vi "太阳能控制器MPPT12.vi"() -> ()   [LabVIEW 2016, in "环境动力监测库.lvlib"]
uses:
  <vilib>/Utility/miscctls.llb/LVPointTypeDef.ctl
  <vilib>/Utility/config.llb/NI_LVConfig.lvlib
  <vilib>/ptbypt/NI_PtbyPt.lvlib
panel:
  out "x+1":u32
  in  "解除告警":bool
  out "串口":string
  in  "串口启用":bool
  in  "报警设置":bool
  in  "MPPT-12 串口":refnum<visa-resource-name> caption="MPPT-12"
  out "状态":string
  out "充放电信息":T1 caption="充放电信息_KWH" {"总累计充电量" format="%.2f"; "当年累计充电量" format="%.2f"; "当月累计充电量" format="%.2f"; "当日累计充电量" format="%.2f"; "当年累计用电量" format="%.2f"; "当月累计用电量" format="%.2f"; "当日累计用电量" format="%.2f"}
  out "通信":bool=TRUE
  out "控制器信息":cluster{"设备温度":dbl}
  out "直流负载信息":cluster{"负载电压":dbl, "负载电流":dbl, "负载功率":dbl}
  out "蓄电池信息":T2
  out "阵列信息":cluster{"阵列电压":dbl, "阵列电流":dbl, "发电功率":dbl}
  # "太阳能控制器MPPT-12"
  # "kW·h"
  # "kW·h"
  # "kW·h"
  # "kW·h"
  # "kW·h"
  # "kW·h"
  # "kW·h"
  # "kW·h"
  # "℃"
  # "V"
  # "A"
  # "W"
  # "V"
  # "A"
  # "V"
  # "A"
  # "℃"
  # "%"
  # "V"
  # "A"
  # "W"
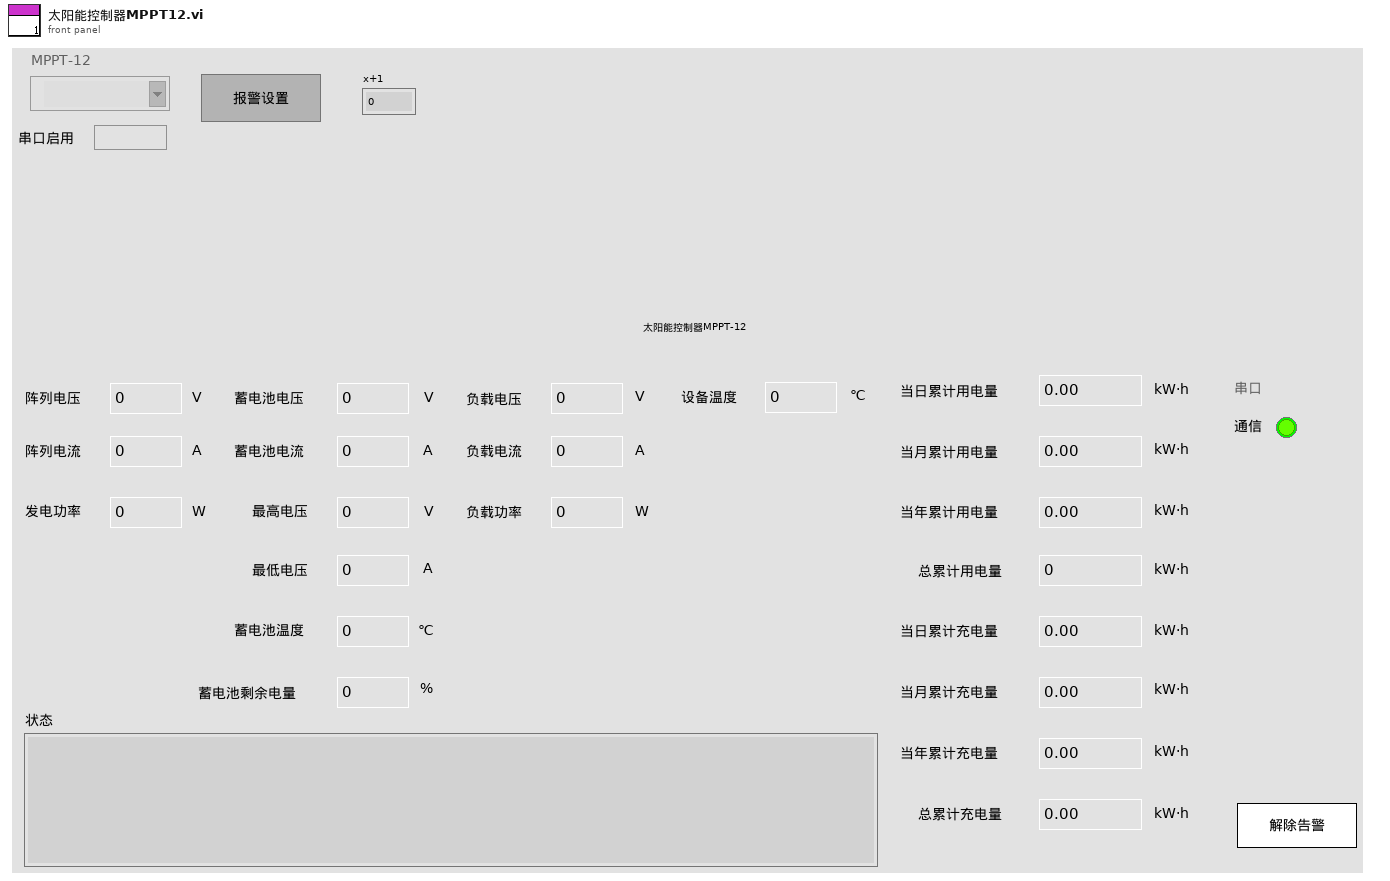
[diagram p1: front panel]
types:
  T1 = cluster{"当日累计用电量":sgl, "当月累计用电量":sgl, "当年累计用电量":sgl, "总累计用电量":sgl, "当日累计充电量":sgl, "当月累计充电量":sgl, "当年累计充电量":sgl, "总累计充电量":sgl}
  T2 = cluster{"蓄电池电压":dbl, "蓄电池电流":dbl, "最高电压":dbl, "最低电压":dbl, "蓄电池温度":dbl, "蓄电池剩余电量":dbl}
  T3 = cluster{"baud rate (bps)":u32, "stop bits":u16, "parity":u16, "flow control":u16, "timeout":u32, "retries":i32}
  T4 = cluster{"监测项描述:输出":string, "连接方式":enum16{"串口", "TCP"}, "端口":string, "IP address:":string, "Port:":string, "站号":u64, "传感器型号":string, "波特率":u64, "data bits":u64, "停止位":u16, "奇偶校验":u16, "声光告警启用":bool}
  T5 = typedef "LVPointTypeDef.ctl" = cluster{"Horizontal":i16, "Vertical":i16}
  T6 = cluster{"漏水监测输出":cluster{"漏水监测告警":bool, "告警内容":string}, "门禁监测输出":cluster{"门禁监测告警":bool, "告警内容":string}, "门禁监测输出2":cluster{"门禁监测告警":bool, "告警内容":string}, "温湿度监测输出":cluster{"温湿度监测告警":bool, "告警内容":string}, "烟雾监测输出":cluster{"烟雾监测告警":bool, "告警内容":string}, "空调监测输出":cluster{"空调监测告警":bool, "告警内容":string}, "自动重合闸输出":cluster{"自动重合闸告警":bool, "告警内容":string}, "红外入侵输出":cluster{"红外入侵告警":bool, "告警内容":string}, "振动输出":cluster{"振动告警":bool, "告警内容":string}, "UPS输出":cluster{"UPS告警":bool, "告警内容":string}, "蓄电池输出":cluster{"蓄电池告警":bool, "告警内容":string}, "蓄电池输出2":cluster{"蓄电池告警":bool, "告警内容":string}, "GPS输出":cluster{"定位告警":bool, "告警内容":string}, "北斗输出":cluster{"定位告警":bool, "告警内容":string}, "气象输出":cluster{"气象告警":bool, "告警内容":string}, "废液输出":cluster{"废液告警":bool, "告警内容":string}, "废液输出2":cluster{"废液告警":bool, "告警内容":string}}
  T7 = cluster{"时间":timestamp, "阵列电压_V":dbl, "阵列电流_A":dbl, "发电功率_W":dbl, "蓄电池电压_V":dbl, "蓄电池电流_A":dbl, "最高电压_V":dbl, "最低电压_A":dbl, "蓄电池温度_℃":dbl, "蓄电池剩余电量_%":dbl, "负载电压_V":dbl, "负载电流_A":dbl, "负载功率_W":dbl, "设备温度_℃":dbl, "当日累计用电量_KWH":dbl, "当月累计用电量_KWH":dbl, "当年累计用电量_KWH":dbl, "总累计用电量_KWH":dbl, "当日累计充电量_KWH":dbl, "当月累计充电量_KWH":dbl, "当年累计充电量_KWH":dbl, "总累计充电量_KWH":dbl}
  T8 = typedef "LVDateTimeRec.ctl" = cluster{"秒数的小数部分":dbl, "秒":i32, "分":i32, "时":i32, "日":i32, "月":i32, "年":i32, "天数（周）":i32, "天数（年）":i32, "DST":i32}
  T9 = cluster{"市电":cluster{"状态":bool, "电压:":u16, "电流：":dbl, "详情  ":bool}, "UPS":cluster{"状态":bool, "输入电压:":sgl, "输出电压:":sgl, "电池电量:":u8, "电量":u16, "详情  ":bool}, "蓄电池12V":cluster{"状态":bool, "电压:":sgl, "电流:":sgl, "电池电量:":u8, "电量":u16, "详情  ":bool}, "蓄电池24V":cluster{"状态":bool, "电压:":sgl, "电流:":sgl, "电池电量:":u8, "电量":u16, "详情  ":bool}}
  T10 = cluster{"状态":cluster{"蓄电池状态":string, "阵列状态":string, "充电状态":string, "负载状态":string, "设备状态":string}, "充放电信息":cluster{"当日累计用电量":sgl, "当月累计用电量":sgl, "当年累计用电量":sgl, "总累计用电量":sgl, "当日累计充电量":sgl, "当月累计充电量":sgl, "当年累计充电量":sgl, "总累计充电量":sgl}, "控制器信息":cluster{"设备温度℃":dbl}, "蓄电池信息":cluster{"蓄电池电压V":dbl, "蓄电池电流A":dbl, "最高电压V":dbl, "最低电压A":dbl, "蓄电池温度℃":dbl, "蓄电池剩余电量%":dbl}, "阵列信息":cluster{"阵列电压V":dbl, "阵列电流A":dbl, "发电功率W":dbl}, "直流负载信息":cluster{"负载电压V":dbl, "负载电流A":dbl, "负载功率W":dbl}, "error out":errorcluster}
  T11 = enum32{"Bad", "Idle", "Run top level", "Running"}
  T12 = typedef "NI_LVConfig.lvlib/Config Data RefNum.ctl" = refnum<k1>
  T13 = enum8{"Enabled", "Disabled", "Disabled and Grayed Out"}
  T14 = cluster{"蓄电池电压V":dbl, "蓄电池电流A":dbl, "最高电压V":dbl, "最低电压A":dbl, "蓄电池温度℃":dbl, "蓄电池剩余电量%":dbl}
  T15 = cluster{"蓄电池状态":string, "阵列状态":string, "充电状态":string, "负载状态":string, "设备状态":string}
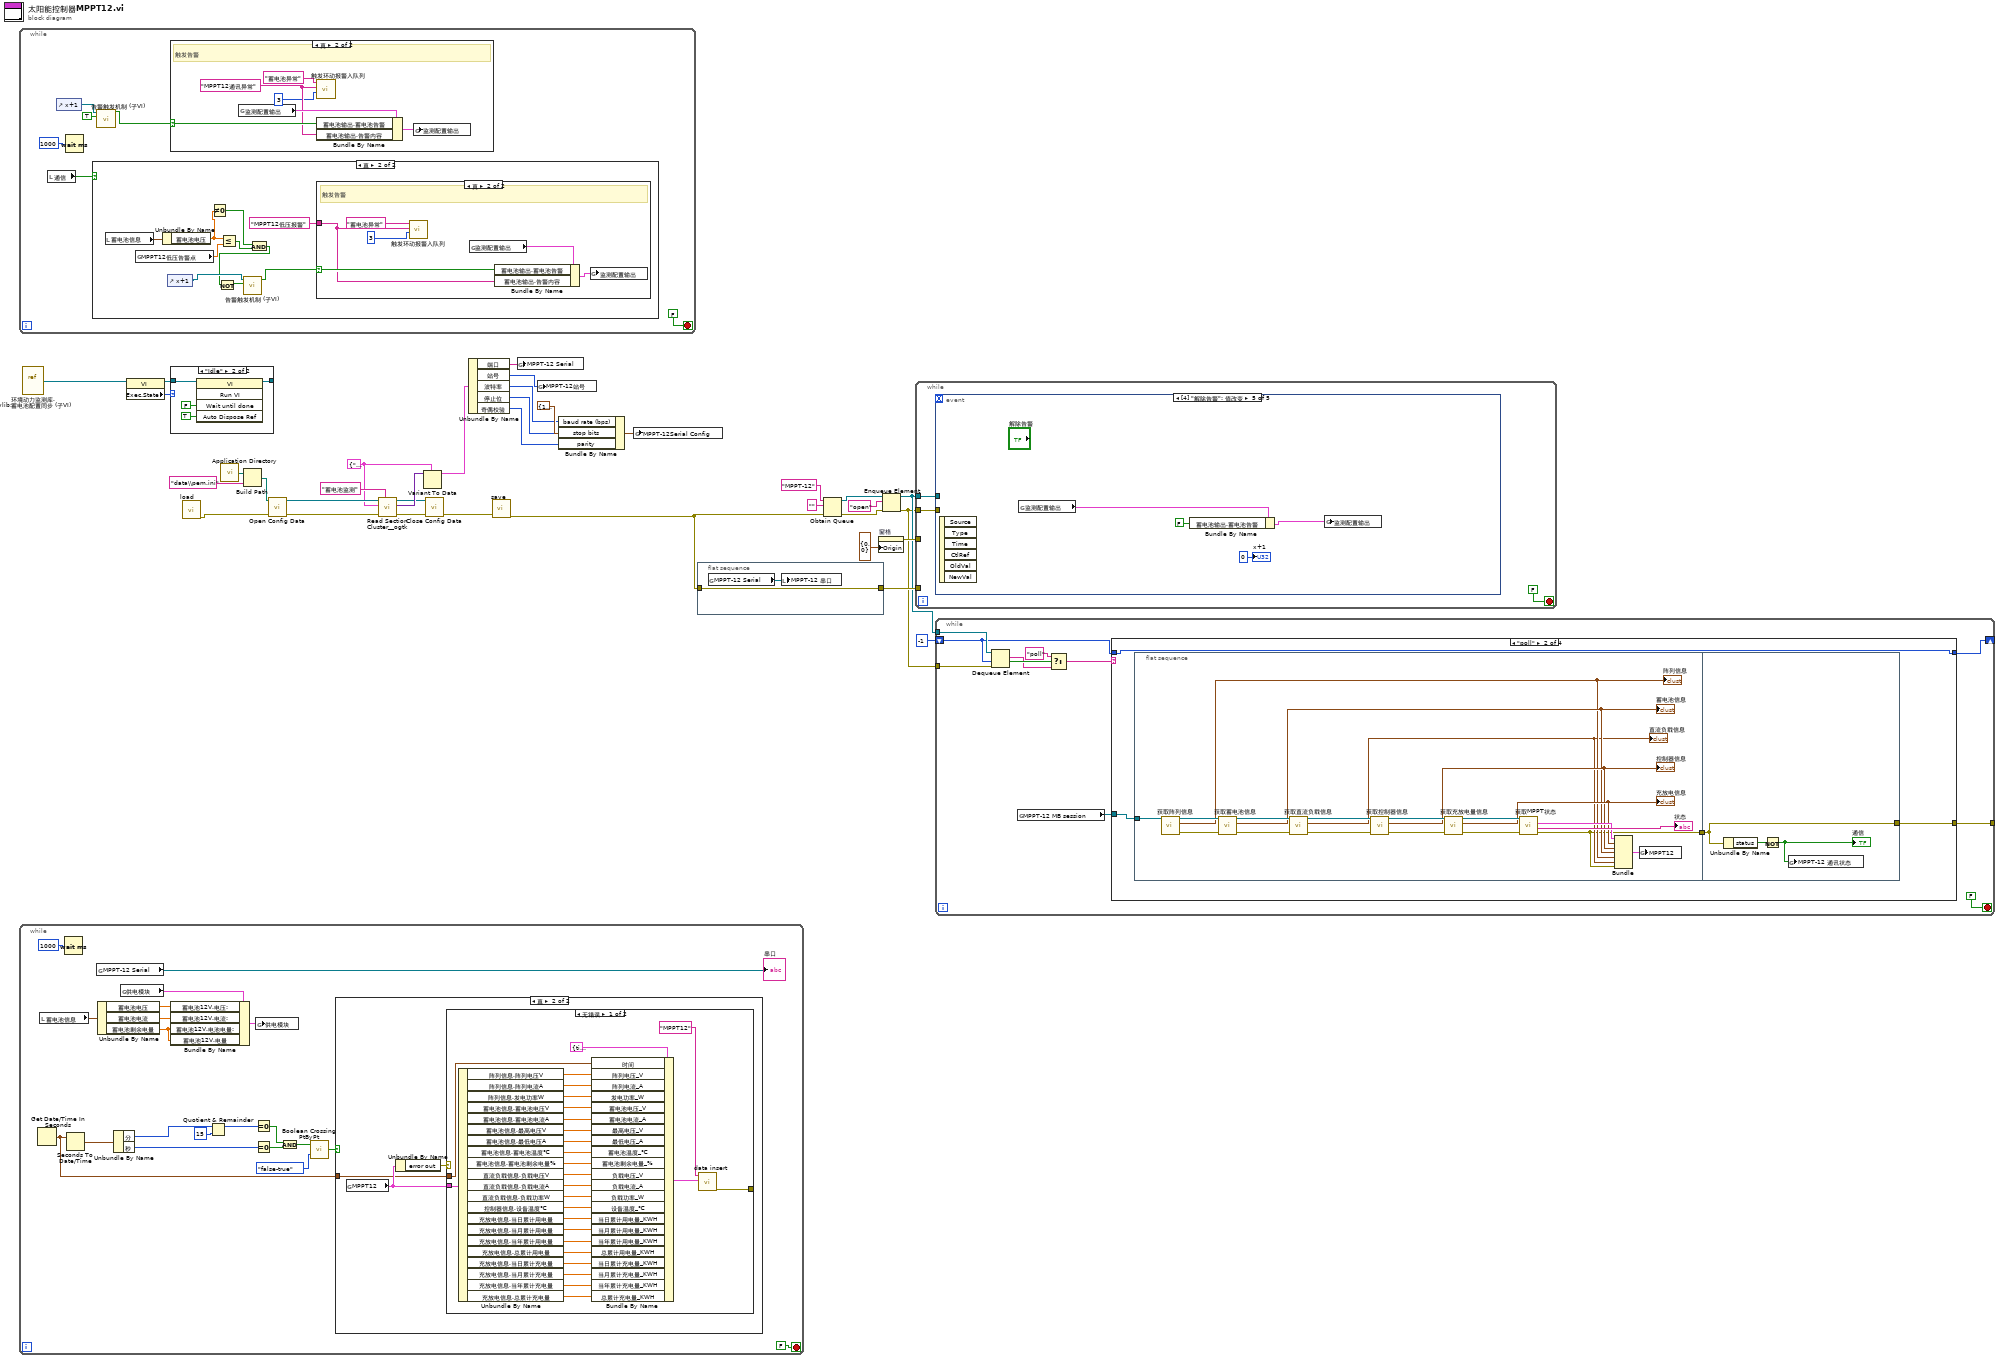
[diagram p0: block diagram]
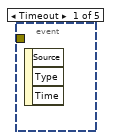
[diagram p8: hidden frame]
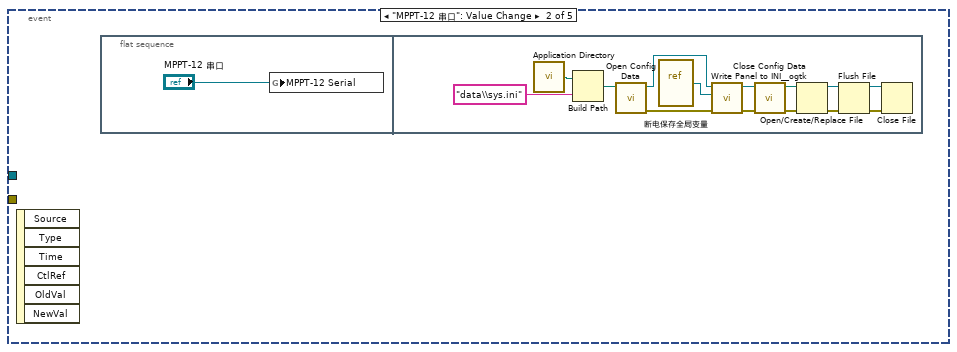
[diagram p9: hidden frame]
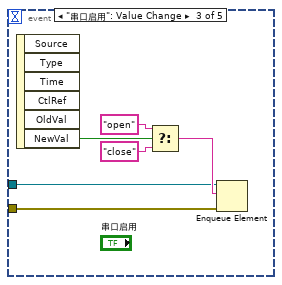
[diagram p10: hidden frame]
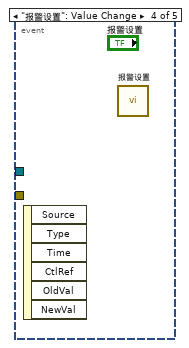
[diagram p11: hidden frame]
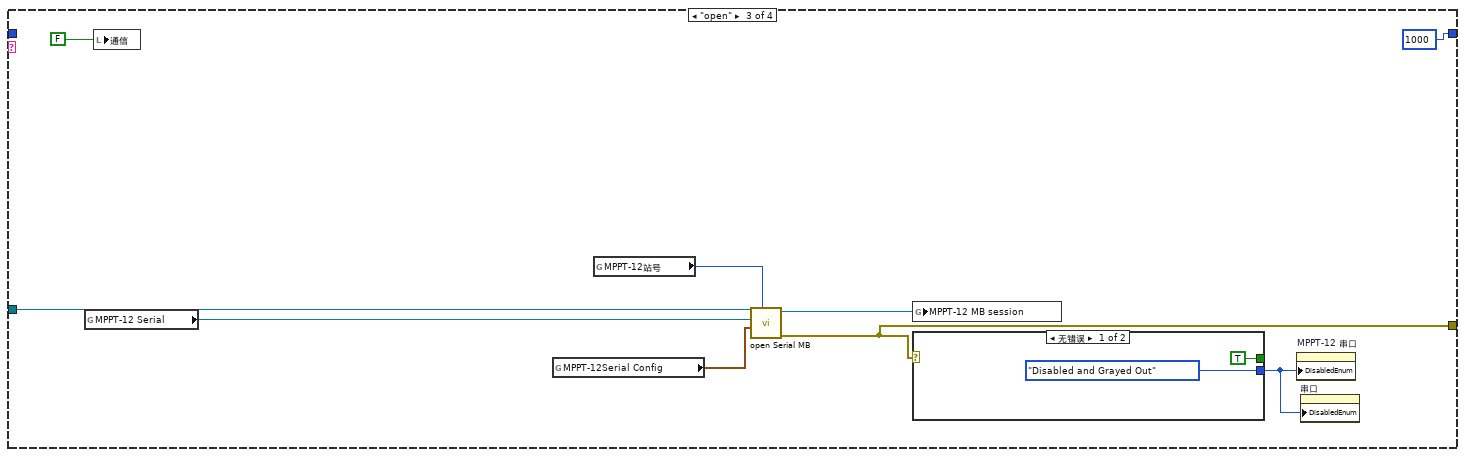
[diagram p13: hidden frame]
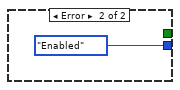
[diagram p14: hidden frame]
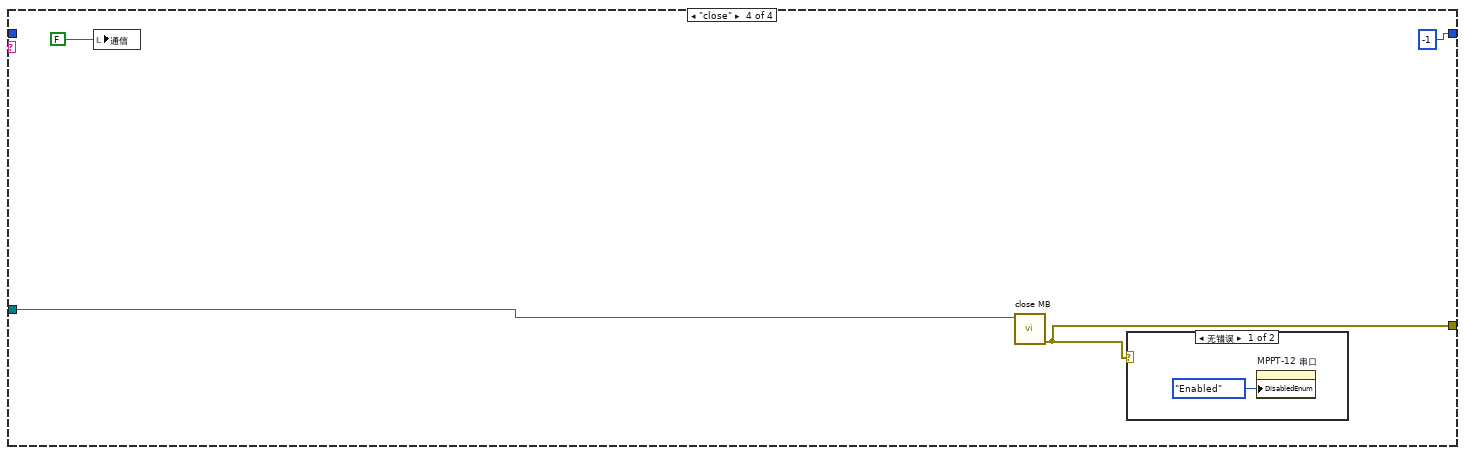
[diagram p15: hidden frame]
diagram:
  w14 = T4 {"监测项描述:输出"="", "连接方式"=enum."串口", "端口"="", "IP address:"="", "Port:"="", "站号"=19200, "传感器型号"="", "波特率"=19200, "data bits"=8, "停止位"=10, "奇偶校验"=0, "声光告警启用"=FALSE} ("输入簇")
  n1 = while {
    stop <- FALSE stop-if-true
    n2 = local read "通信"() -> (w39:bool)
    n3 = control-ref of="x+1"() -> (w38:refnum<vi>)
    n4 = Wait (ms)(milliseconds to wait=u32 1000 ("等待时间（毫秒）")) -> ()  [unwired: 1 out]
    n5 = case shown="真" w39 {
      frame False {
      }
      frame True {
        n6 = local read "蓄电池信息"() -> (w57:T2)
        n7 = global read "断电保存全局变量.vi" "MPPT12低压告警点"() -> (w56:dbl)
        n8 = Unbundle By Name(w57) -> ("蓄电池电压"=w50:dbl)
        n9 = control-ref of="x+1"() -> (w52:refnum<vi>)
        n10 = Not Equal To 0?(x=w50) -> (x != 0?=w49:bool)
        n11 = Less Or Equal?(x=w50, y=w56) -> (x <= y?=w51:bool)
        n12 = And(x=w49, y=w51) -> (x .and. y?=w48:bool)
        n13 = Not(x=w48) -> (.not. x?=w54:bool)
        n14 = call "告警触发机制 (子VI).vi"("状态输出"=w54, "Digital输入"=w52) -> ("触发告警"=w53:bool)  [unwired: 8 in, 1 out]
        n15 = case shown="真" w53 {
          selector: w53 -> [_ w63]
          tunnel: "MPPT12低压报警" ("设备") -> [_ w59]
          frame False {
          }
          frame True {
            # "触发告警"
            n16 = call "触发环动报警入队列.vi"("code"=3, "备注"=w59, "报警内容"="蓄电池异常" ("设备")) -> ()  [unwired: 9 in]
            n17 = global read "内部交互全局变量.vi" "监测配置输出"() -> (w62:T6)
            n18 = Bundle By Name(cluster=w62, "蓄电池输出.蓄电池告警"=w63, "蓄电池输出.告警内容"=w59) -> (w61:T6)
            n19 = global write "内部交互全局变量.vi" "监测配置输出"(w61) -> ()
          }
        }
      }
    }
    n20 = call "告警触发机制 (子VI).vi"("状态输出"=TRUE, "Digital输入"=w38) -> ("触发告警"=w37:bool)  [unwired: 8 in, 1 out]
    n21 = case shown="真" w37 {
      selector: w37 -> [_ w47]
      frame False {
      }
      frame True {
        w43 = "MPPT12通讯异常" ("报警内容")
        # "触发告警"
        n22 = global read "内部交互全局变量.vi" "监测配置输出"() -> (w46:T6)
        n23 = call "触发环动报警入队列.vi"("code"=3, "备注"=w43, "报警内容"="蓄电池异常" ("设备")) -> ()  [unwired: 9 in]
        n24 = Bundle By Name(cluster=w46, "蓄电池输出.蓄电池告警"=w47, "蓄电池输出.告警内容"=w43) -> (w45:T6)
        n25 = global write "内部交互全局变量.vi" "监测配置输出"(w45) -> ()
      }
    }
  }
  n26 = while {
    stop <- FALSE stop-if-true
    n27 = Get Date/Time In Seconds() -> (seconds since 1Jan1904=w71:timestamp)
    n28 = local read "蓄电池信息"() -> (w67:T2)
    n29 = Wait (ms)(milliseconds to wait=u32 1000 ("等待时间（毫秒）")) -> ()  [unwired: 1 out]
    n30 = Seconds To Date/Time(time stamp (now)=w71) -> (date time rec=w81:T8)  [unwired: 1 in]
    n31 = global read "断电保存全局变量.vi" "MPPT-12 Serial"() -> (→"串口":refnum<visa-resource-name>)
    n32 = Unbundle By Name(w67) -> ("蓄电池电压"=w66:dbl, "蓄电池电流"=w65:dbl, "蓄电池剩余电量"=w64:dbl)
    n33 = Unbundle By Name(w81) -> ("分"=w80:i32, "秒"=w77:i32)
    n34 = global read "内部交互全局变量.vi" "供电模块"() -> (w69:T9)
    n35 = Bundle By Name(cluster=w69, "蓄电池12V.电压:"=w66, "蓄电池12V.电流:"=w65, "蓄电池12V.电池电量:"=w64, "蓄电池12V.电量"=w64) -> (w68:T9)
    n36 = Quotient & Remainder(x=w80, y=15) -> (x-y*floor(x/y)=w78:i32)  [unwired: 1 out]
    n37 = Equal To 0?(x=w78) -> (x = 0?=w76:bool)
    n38 = Equal To 0?(x=w77) -> (x = 0?=w75:bool)
    n39 = global write "内部交互全局变量.vi" "供电模块"(w68) -> ()
    n40 = And(x=w76, y=w75) -> (x .and. y?=w74:bool)
    n41 = call <vilib>:"Boolean Crossing PtByPt.vi"("direction"=enum16{"either", "false-true", "true-false"}."false-true", "input"=w74) -> ("crossing"=w72:bool)  [unwired: 1 in]
    n42 = case shown="真" w72 {
      tunnel: w71 -> [_ w84]
      frame False {
      }
      frame True {
        n43 = global read "太阳能控制器全局.vi" "MPPT12"() -> (w85:T10)
        n44 = Unbundle By Name(w85) -> ("error out"=w86:errorcluster)
        n45 = case shown="无错误" w86 {
          tunnel: w85 -> [w91 _]
          tunnel: w84 -> [w90 _]
          tunnel: [w87 _] -> _
          frame No Error {
            n46 = Unbundle By Name(w91) -> ("阵列信息.阵列电压V"=w93:dbl, "阵列信息.阵列电流A"=w94:dbl, "阵列信息.发电功率W"=w95:dbl, "蓄电池信息.蓄电池电压V"=w96:dbl, "蓄电池信息.蓄电池电流A"=w97:dbl, "蓄电池信息.最高电压V"=w98:dbl, "蓄电池信息.最低电压A"=w99:dbl, "蓄电池信息.蓄电池温度℃"=w100:dbl, "蓄电池信息.蓄电池剩余电量%"=w101:dbl, "直流负载信息.负载电压V"=w102:dbl, "直流负载信息.负载电流A"=w103:dbl, "直流负载信息.负载功率W"=w104:dbl, "控制器信息.设备温度℃"=w105:dbl, "充放电信息.当日累计用电量"=w106:sgl, "充放电信息.当月累计用电量"=w107:sgl, "充放电信息.当年累计用电量"=w108:sgl, "充放电信息.总累计用电量"=w109:sgl, "充放电信息.当日累计充电量"=w110:sgl, "充放电信息.当月累计充电量"=w111:sgl, "充放电信息.当年累计充电量"=w112:sgl, "充放电信息.总累计充电量"=w113:sgl)
            n47 = Bundle By Name(cluster=T7 {"时间"=timestamp(0 s since 1904-01-01), "阵列电压_V"=0.0, "阵列电流_A"=0.0, "发电功率_W"=0.0, "蓄电池电压_V"=0.0, "蓄电池电流_A"=0.0, "最高电压_V"=0.0, "最低电压_A"=0.0, "蓄电池温度_℃"=0.0, "蓄电池剩余电量_%"=0.0, "负载电压_V"=0.0, "负载电流_A"=0.0, "负载功率_W"=0.0, "设备温度_℃"=0.0, "当日累计用电量_KWH"=0.0, "当月累计用电量_KWH"=0.0, "当年累计用电量_KWH"=0.0, "总累计用电量_KWH"=0.0, "当日累计充电量_KWH"=0.0, "当月累计充电量_KWH"=0.0, "当年累计充电量_KWH"=0.0, "总累计充电量_KWH"=0.0} ("data in"), "时间"=w90, "阵列电压_V"=w93, "阵列电流_A"=w94, "发电功率_W"=w95, "蓄电池电压_V"=w96, "蓄电池电流_A"=w97, "最高电压_V"=w98, "最低电压_A"=w99, "蓄电池温度_℃"=w100, "蓄电池剩余电量_%"=w101, "负载电压_V"=w102, "负载电流_A"=w103, "负载功率_W"=w104, "设备温度_℃"=w105, "当日累计用电量_KWH"=w106, "当月累计用电量_KWH"=w107, "当年累计用电量_KWH"=w108, "总累计用电量_KWH"=w109, "当日累计充电量_KWH"=w110, "当月累计充电量_KWH"=w111, "当年累计充电量_KWH"=w112, "总累计充电量_KWH"=w113) -> (w89:T7)
            n48 = call "data insert.vi"("data in"=w89, "table"="MPPT12") -> ("error out"=w87:errorcluster)  [unwired: 9 in]
          }
          frame Error {
          }
        }
      }
    }
  }
  n49 = vi-ref "环境动力监测库.lvlib:蓄电池配置同步 (子VI).vi"() -> (w10:refnum<vi>)
  n50 = property class="VI"(reference=w10) -> (reference out=w11:refnum<vi>, "Exec.State"=w12:T11)  [unwired: 1 in, 1 out]
  n51 = case shown="\"Idle\"" w12 {
    tunnel: w11 -> [w114 w116]
    tunnel: [w114 w115] -> _
    frame "Bad", Default {
    }
    frame "Idle" {
      n52 = invoke class="VI" method="Run VI"(reference=w116, "Wait until done"=FALSE ("结束前等待"), "Auto Dispose Ref"=TRUE ("自动销毁引用")) -> (reference out=w115:refnum<vi>)  [unwired: 2 in, 4 out]
    }
  }
  n53 = call "load.vi"() -> ("error out"=w3:errorcluster)  [unwired: 11 in]
  n54 = call <vilib>:"Application Directory.vi"() -> ("Application Directory"=w18:path)
  n55 = Build Path(base path=w18, name or relative path="data\\pem.ini" ("名称或相对路径")) -> (appended path=w17:path)
  n56 = call <vilib>:"Open Config Data.vi"("error in (no error)"=w3, "configuration file path"=w17) -> ("error out"=w16:errorcluster, "refnum"=w15:T12)  [unwired: 7 in, 1 out]
  n57 = call <userlib>:"Read Section Cluster__ogtk.vi"("section (optional)"="蓄电池监测", "error in (no error)"=w16, "Section Formatted Cluster Type"=w14, "refnum"=w15) -> ("error out"=w22:errorcluster, "Section Formatted Cluster"=w23:variant, "dup refnum"=w21:T12)  [unwired: 3 in, 2 out]
  n58 = Variant To Data(type=w14, Variant=w23) -> (data=w24:T4)  [unwired: 1 in, 1 out]
  n59 = call <vilib>:"Close Config Data.vi"("error in (no error)"=w22, "refnum"=w21) -> ("error out"=w2:errorcluster)  [unwired: 8 in, 1 out]
  n60 = Unbundle By Name(w24) -> ("端口"=w13:string, "站号"=w7:u64, "波特率"=w6:u64, "停止位"=w5:u16, "奇偶校验"=w4:u16)
  n61 = call "save.vi"("error in (no error)"=w2) -> ("error out"=w1:errorcluster)  [unwired: 10 in]
  n62 = global write "断电保存全局变量.vi" "MPPT-12 Serial"(w13) -> ()
  n63 = global write "断电保存全局变量.vi" "MPPT-12站号"(w7) -> ()
  n64 = Bundle By Name(cluster=T3 {"baud rate (bps)"=115200, "stop bits"=10, "parity"=0, "flow control"=0, "timeout"=1000, "retries"=1} ("MPPT-24Serial Config"), "baud rate (bps)"=w6, "stop bits"=w5, "parity"=w4) -> (w8:T3)
  n65 = global write "断电保存全局变量.vi" "MPPT-12Serial Config"(w8) -> ()
  n66 = flat-sequence {
    tunnel: w1 -> [w119]
    tunnel: [w119] -> w27
    frame #0 {
      n67 = global read "断电保存全局变量.vi" "MPPT-12 Serial"() -> (w120:refnum<visa-resource-name>)
      n68 = local write "MPPT-12 串口"(w120) -> ()
    }
  }
  n69 = Obtain Queue(name (unnamed)="MPPT-12" ("名称（未命名）"), element data type="", error in (no error)=w1) -> (queue out=w29:refnum<queue>, error out=w28:errorcluster)  [unwired: 2 in, 1 out]
  n70 = property on="窗格" class="Pane"("Origin"=T5 {"Horizontal"=0, "Vertical"=0} ("原点")) -> (error out=w33:errorcluster)  [unwired: 2 in, 1 out]
  n71 = Enqueue Element(queue=w29, element="open" ("元素"), error in (no error)=w28) -> (queue out=w26:refnum<queue>, error out=w25:errorcluster)  [unwired: 1 in, 1 out]
  n72 = while {
    tunnel: w33 -> [_]
    tunnel: w27 -> [_]
    tunnel: w26 -> [w122]
    tunnel: w25 -> [w121]
    stop <- FALSE stop-if-true
    n73 = event shown="[4] \"解除告警\": 值改变" {
      selector: _ -> [_ _ _ _ _]
      dyn-events: _ -> [_ _ _ _ _]
      timeout: _ -> [_ _ _ _ _]
      tunnel: w122 -> [_ _ w140 _ _]
      tunnel: w121 -> [_ _ w139 _ _]
      event Timeout {
        n74 = event-data() -> ()  [unwired: 1 in, 3 out]
      }
      event "MPPT-12 串口": Value Change {
        n75 = event-data() -> ()  [unwired: 1 in, 6 out]
        n76 = flat-sequence {
          frame #0 {
            n77 = global write "断电保存全局变量.vi" "MPPT-12 Serial"("MPPT-12 串口") -> ()
          }
          frame #1 {
            n78 = call <vilib>:"Application Directory.vi"() -> ("Application Directory"=w138:path)
            n79 = Build Path(base path=w138, name or relative path="data\\sys.ini" ("名称或相对路径")) -> (appended path=w136:path)
            n80 = call <vilib>:"Open Config Data.vi"("configuration file path"=w136) -> ("error out"=w132:errorcluster, "refnum"=w135:T12)  [unwired: 8 in, 1 out]
            n81 = vi-ref "断电保存全局变量.vi"() -> (w134:refnum<vi>)
            n82 = call <userlib>:"Write Panel to INI__ogtk.vi"("error in (no error)"=w132, "VI ref"=w134, "refnum"=w135) -> ("error out"=w131:errorcluster, "refnum out"=w133:T12)  [unwired: 7 in]
            n83 = call <vilib>:"Close Config Data.vi"("error in (no error)"=w131, "refnum"=w133) -> ("error out"=w126:errorcluster, "file path"=w125:path)  [unwired: 8 in]
            n84 = Open/Create/Replace File(file path (use dialog)=w125, error in=w126) -> (refnum out=w129:refnum<file>, error out=w130:errorcluster)  [unwired: 4 in, 1 out]
            n85 = Flush File(refnum=w129, error in=w130) -> (refnum out=w128:refnum<file>, error out=w127:errorcluster)
            n86 = Close File(refnum=w128, error in=w127) -> ()  [unwired: 2 out]
          }
        }
      }
      event "串口启用": Value Change {
        n87 = event-data() -> ("NewVal"=w141:bool)  [unwired: 1 in, 5 out]
        n88 = Select(t="open", s=w141, f="close") -> (s? t:f=w143:string)
        n89 = Enqueue Element(queue=w140, element=w143, error in (no error)=w139) -> ()  [unwired: 1 in, 3 out]
      }
      event "报警设置": Value Change {
        n90 = event-data() -> ()  [unwired: 1 in, 6 out]
        n91 = call "报警设置.vi"() -> ()  [unwired: 12 in]
      }
      event "解除告警": Value Change {
        n92 = event-data() -> ()  [unwired: 1 in, 6 out]
        n93 = global read "内部交互全局变量.vi" "监测配置输出"() -> (w146:T6)
        n94 = Bundle By Name(cluster=w146, "蓄电池输出.蓄电池告警"=FALSE) -> (w145:T6)
        n95 = global write "内部交互全局变量.vi" "监测配置输出"(w145) -> ()
        "x+1" <- u32 0 ("x+1")
      }
    }
  }
  n96 = while {
    shift-right: [w150] -> _
    shift-left: -1 ("超时毫秒(-1)") -> [w151]
    tunnel: w26 -> [w156]
    tunnel: [w152] -> _
    tunnel: w25 -> [w149]
    stop <- FALSE stop-if-true
    n97 = Dequeue Element(queue=w156, timeout in ms (-1)=w151, error in (no error)=w149) -> (element=w157:string, timed out?=w159:bool)  [unwired: 2 out]
    n98 = global read "太阳能控制器全局.vi" "MPPT-12 MB session"() -> (w153:refnum<class "MB_Master.lvclass">)
    n99 = Select(t="poll" ("元素"), s=w159, f=w157) -> (s? t:f=w154:string)
    n100 = case shown="\"poll\"" w154 {
      tunnel: w153 -> [_ w164 w195 w202]
      tunnel: [_ w162 w193 w200] -> w152
      tunnel: w151 -> [w160 w161 _ _]
      tunnel: [w160 w161 1000 ("超时毫秒(-1)") -1 ("超时毫秒(-1)")] -> w150
      frame Default {
      }
      frame "poll" {
        n101 = flat-sequence {
          tunnel: w164 -> [w184]
          tunnel: [w166] -> w163
          tunnel: w163 -> [w185]
          tunnel: [w185] -> w162
          frame #0 {
            n102 = call "获取阵列信息.vi"("MB session in"=w184) -> ("error out"=w182:errorcluster, "阵列信息"=w168:cluster{"阵列电压V":dbl, "阵列电流A":dbl, "发电功率W":dbl}, "MB session out"=w183:refnum<class "MB_Master.lvclass">)  [unwired: 8 in]
            "阵列信息" <- w168
            n103 = call "获取蓄电池信息.vi"("error in (no error)"=w182, "MB session in"=w183) -> ("error out"=w180:errorcluster, "蓄电池信息"=w169:T14, "MB session out"=w181:refnum<class "MB_Master.lvclass">)  [unwired: 7 in]
            "蓄电池信息" <- w169
            n104 = call "获取直流负载信息.vi"("error in (no error)"=w180, "MB session in"=w181) -> ("error out"=w178:errorcluster, "直流负载信息"=w167:cluster{"负载电压V":dbl, "负载电流A":dbl, "负载功率W":dbl}, "MB session out"=w179:refnum<class "MB_Master.lvclass">)  [unwired: 7 in]
            "直流负载信息" <- w167
            n105 = call "获取控制器信息.vi"("error in (no error)"=w178, "MB session in"=w179) -> ("error out"=w176:errorcluster, "控制器信息"=w170:cluster{"设备温度℃":dbl}, "MB session out"=w177:refnum<class "MB_Master.lvclass">)  [unwired: 7 in]
            "控制器信息" <- w170
            n106 = call "获取充放电量信息.vi"("error in (no error)"=w176, "MB session in"=w177) -> ("error out"=w174:errorcluster, "充放电信息"=w171:T1, "MB session out"=w175:refnum<class "MB_Master.lvclass">)  [unwired: 7 in]
            "充放电信息" <- w171
            n107 = call "获取MPPT状态.vi"("error in (no error)"=w174, "MB session in"=w175) -> ("error out"=w166:errorcluster, "结果字符串"=→"状态":string, "状态"=w172:T15)  [unwired: 6 in, 1 out]
            n108 = Bundle("状态"=w172, "充放电信息"=w171, "控制器信息"=w170, "蓄电池信息"=w169, "阵列信息"=w168, "直流负载信息"=w167, "error out"=w166) -> (w165:T10)  [unwired: 1 in]
            n109 = global write "太阳能控制器全局.vi" "MPPT12"(w165) -> ()
          }
          frame #1 {
            n110 = Unbundle By Name(w185) -> ("status"=w187:bool)
            n111 = Not(x=w187) -> (.not. x?=w186:bool)
            "通信" <- w186
            n112 = global write "太阳能控制器全局.vi" "MPPT-12 通讯状态"(w186) -> ()
          }
        }
      }
      frame "open" {
        n113 = global read "断电保存全局变量.vi" "MPPT-12 Serial"() -> (w191:refnum<visa-resource-name>)
        n114 = local write "通信"(FALSE ("通讯状态 2")) -> ()
        n115 = global read "断电保存全局变量.vi" "MPPT-12Serial Config"() -> (w188:T3)
        n116 = global read "断电保存全局变量.vi" "MPPT-12站号"() -> (w189:u64)
        n117 = call "open Serial MB.vi"("Slave ID"=w189, "Serial Config"=w188, "VISA Resource"=w191, "MB session in"=w195) -> ("error out"=w193:errorcluster, "MB session out"=w194:refnum<class "MB_Master.lvclass">)  [unwired: 6 in]
        n118 = global write "太阳能控制器全局.vi" "MPPT-12 MB session"(w194) -> ()
        n119 = case shown="无错误" w193 {
          tunnel: [T13."Disabled and Grayed Out" ("禁用") T13."Enabled" ("禁用")] -> w190
          tunnel: [TRUE _] -> _
          frame No Error {
          }
          frame Error {
          }
        }
        n120 = property on="MPPT-12 串口" class="VISAName"("DisabledEnum"=w190) -> ()  [unwired: 2 in, 2 out]
        n121 = property on="串口" class="Str"("DisabledEnum"=w190) -> ()  [unwired: 2 in, 2 out]
      }
      frame "close" {
        n122 = local write "通信"(FALSE ("通讯状态 2")) -> ()
        n123 = call "close MB.vi"("MB session in"=w202) -> ("error out"=w200:errorcluster)  [unwired: 10 in]
        n124 = case shown="无错误" w200 {
          frame No Error {
            n125 = property on="MPPT-12 串口" class="VISAName"("DisabledEnum"=T13."Enabled" ("禁用")) -> ()  [unwired: 2 in, 2 out]
          }
          frame Error {
          }
        }
      }
    }
  }
